vi "Run 02.vi"   [LabVIEW 2016]
uses:
  <vilib>/NXT/Block Support/NXT_ButtonSelector.ctl
  <vilib>/NXT/Dual Mode Library/Waits/Wait_Btn_Press.vi
types:
  T1 = typedef "NXT_ButtonSelector.ctl" = u16
  T2 = typedef "LVHSConnector.ctl" = refnum<class "BrickReference.lvclass">
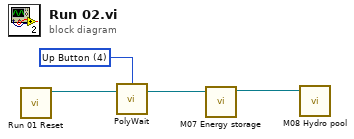
[diagram p0: block diagram]
diagram:
  w4 = T1 4 items=["Enter button"=3, "Left button"=2, "Right button"=1, "Up Button"=4, "Down Button"=5] ("Button (Enter button)")
  n1 = call "Run 01 Reset.vi"() -> ("NXT/EV3 out"=w3:T2)  [unwired: 11 in]
  n2 = call-poly <vilib>:"PolyWait.vi"("NXT/EV3"=w3, "Button (Enter button)"=w4) -> ("NXT/EV3"=w2:T2)  [unwired: 2 in]
  n3 = call "M07 Energy storage.vi"("NXT/EV3"=w2) -> ("EV3 out"=w1:T2)  [unwired: 10 in]
  n4 = call "M08 Hydro pool.vi"("EV3 in"=w1) -> ()  [unwired: 11 in]
